vi "Close.Fpga.vi"(8 "error in (no error)":errorcluster, 11 "FpgaRunner in":refnum<class "FpgaRunner.lvclass">) -> (0 "error out":errorcluster, 3 "FpgaRunner out":refnum<class "FpgaRunner.lvclass">)   [LabVIEW 2020, in "FpgaRunner.lvclass"]
uses:
  FpgaRunner.lvclass
  FpgaRunner.lvclass/FpgaRunner.ctl
  <vilib>/FPGAPlugInAG/Dynamic/niLvFpga_Close_Dynamic.vi
  <vilib>/rvi/interface/nirviCloseFPGA/nirviCloseFPGA.xnode
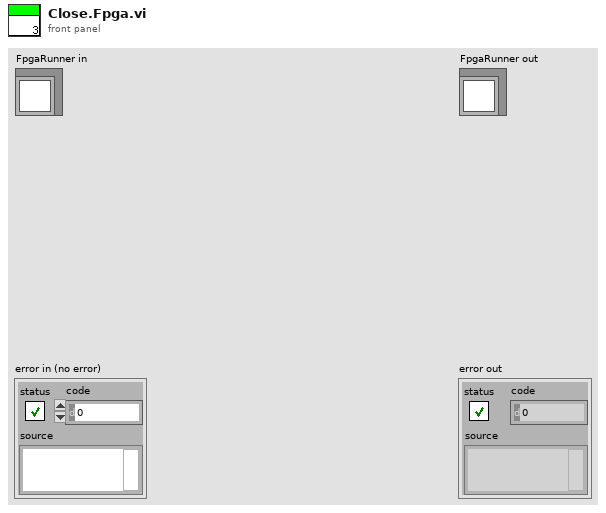
[diagram p1: front panel]
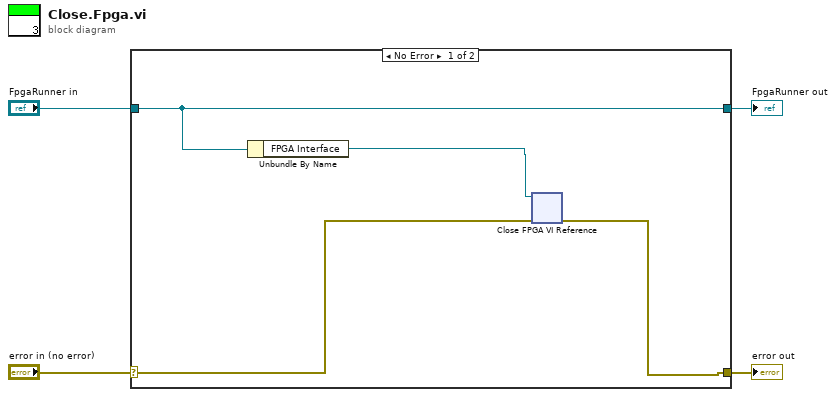
[diagram p0: block diagram]
diagram:
  n1 = case shown="No Error" "error in (no error)" {
    selector: "error in (no error)" -> [w7 w10]
    tunnel: [w8 w10] -> w3
    tunnel: [w6 w9] -> w1
    tunnel: "FpgaRunner in" -> [w6 w9]
    frame No Error {
      n2 = Unbundle By Name(w6) -> ("FPGA Interface"=w5:refnum<k20>)
      n3 = xnode "Close FPGA VI Reference"("FPGA VI Reference In"=w5, "error in"=w7) -> ("error out"=w8:errorcluster)
    }
    frame Error {
    }
  }
  "error out" <- w3
  "FpgaRunner out" <- w1
